vi "ContPostProc.vi"(7 "string seq in":string, 8 "Error In":errorcluster, 10 "File Paths":T2={"Local Save Path"=path "\\\\smbhome.uscs.susx.ac.uk\\cv222/Desktop/data", "Newton Save Path"=path "Z:/#Projects/Entanglement/data", "File Name"="test", "LocalSave"=TRUE}, 11 "readout":T1) -> (0 "error out":errorcluster)   [LabVIEW 2019]
uses:
  controls/FilePaths.ctl
  controls/GlobalExp.vi
  Global.lvlib
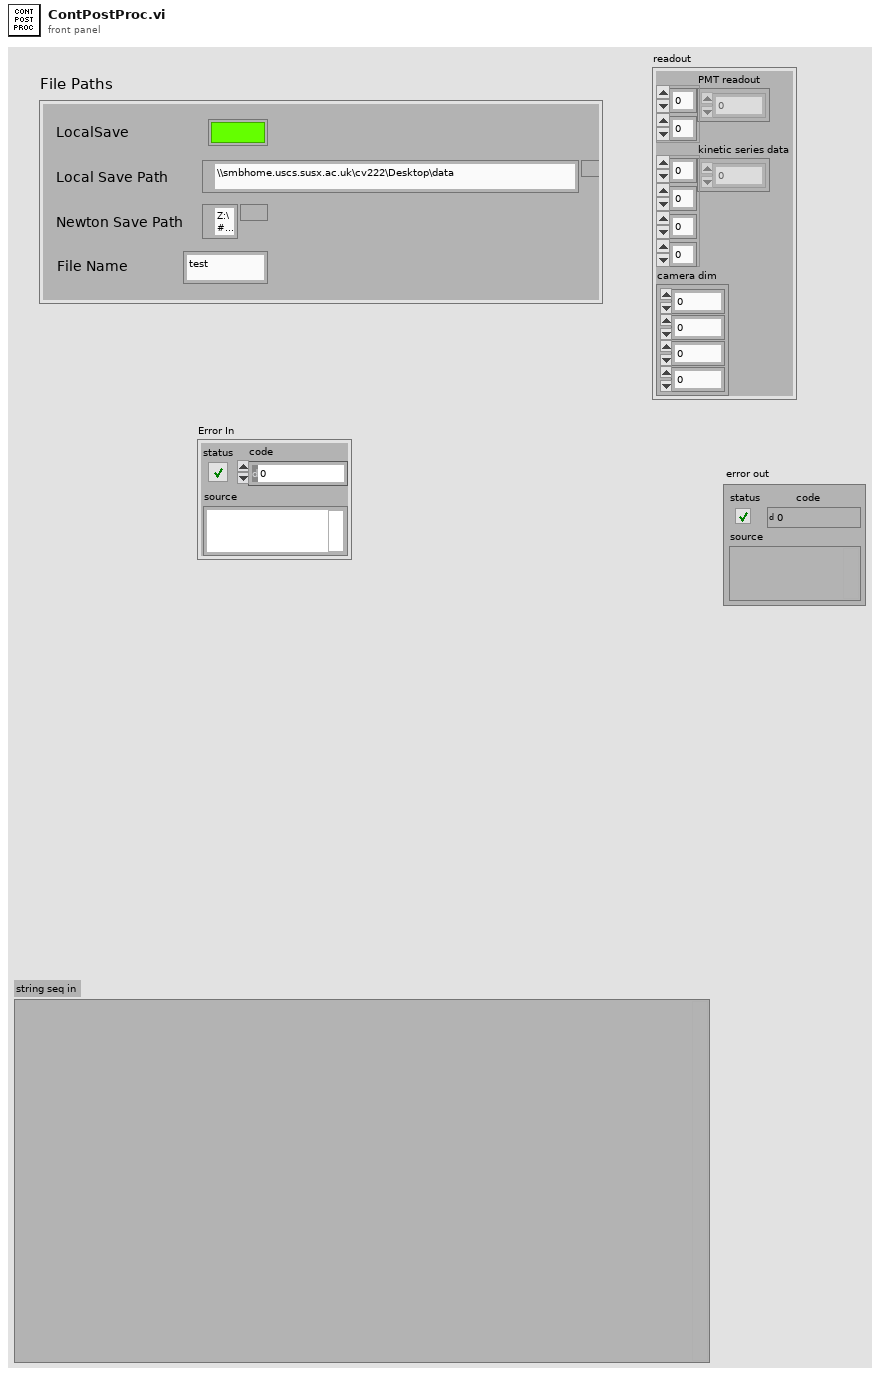
[diagram p1: front panel]
types:
  T1 = cluster{"PMT readout":i16[][], "kinetic series data":i16[][][][], "camera dim":cluster{i32, i32, i32, i32}}
  T2 = typedef "FilePaths.ctl" = cluster{"Local Save Path":path, "Newton Save Path":path, "File Name":string, "LocalSave":bool}
  T3 = typedef "MasterExpControl.ctl" = cluster{"Main Steps":dbl, "Main Runs":dbl, "ExpStatus":enum16{"Innit", "Stop", "Idle", "MainRunning", "AuxRunning"}, "Main Current Step":dbl, "ExpNum":dbl, "NewData":bool, "date":string, "command":string, "Stop":bool, "Pause":bool, "Mathematica":string, "Main/Meta":bool, "UpdateMath":bool, "Camera":bool, "MetaExpOver":bool, "NextMetaExp":bool}
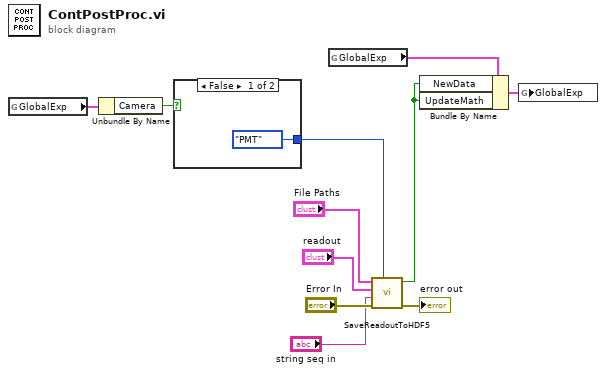
[diagram p0: block diagram]
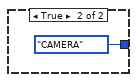
[diagram p2: hidden frame]
diagram:
  n1 = global read "GlobalExp.vi" "GlobalExp"() -> (w6:T3)
  n2 = Unbundle By Name(w6) -> ("Camera"=w3:bool)
  n3 = case shown="False" w3 {
    tunnel: [enum16{"CAMERA", "PMT"}."PMT" ("det_hardware") enum16{"CAMERA", "PMT"}."CAMERA" ("det_hardware")] -> w2
    frame False {
    }
    frame True {
    }
  }
  n4 = global read "GlobalExp.vi" "GlobalExp"() -> (w11:T3)
  n5 = call "SaveReadoutToHDF5.vi"("det_hardware"=w2, "error in"="Error In", "string seq in"="string seq in", "readout"="readout", "File Paths"="File Paths") -> ("error out"=→"error out":errorcluster, "New data?"=w8:bool)  [unwired: 5 in]
  n6 = Bundle By Name(cluster=w11, "NewData"=w8, "UpdateMath"=w8) -> (w10:T3)
  n7 = global write "GlobalExp.vi" "GlobalExp"(w10) -> ()
